vi "ProcesaDatos.vi"() -> ()   [LabVIEW 2010]
uses:
  <vilib>/Utility/file.llb/Write To Spreadsheet File (DBL).vi
panel:
  in  "Stimuli Offset":dbl=0.8
  out "rpm":dbl[](graph)=[-2.67, 1577.33, 1763.996667, 1773.996667, 1763.996667, 1770.663333, 1767.33, 1770.663333, 1770.663333, 1767.33, 1773.996667, 710.6633330000001, 39.350201999999996, -2.67, -2.67, -2.67, -2.67, -2.67, -2.67, -2.67]
  out "u_control":dbl[][](graph)=[[1.8699999999999999, 1.8699999999999999, 1.8699999999999999, 1.8699999999999999, 1.8699999999999999, 1.8699999999999999, 1.8699999999999999, 1.8699999999999999, 1.8699999999999999, 1.8699999999999999, -0.010000000000000009, -0.010000000000000009, -0.010000000000000009, -0.010000000000000009, -0.010000000000000009, -0.010000000000000009, -0.010000000000000009, -0.010000000000000009, -0.010000000000000009, -0.010000000000000009]]
  in  "Done":bool
  out "Signals":dbl[][](graph)=[[0.79, 0.79, 0.79, 0.79, 0.79, 0.79, 0.79, 0.79, 0.79, 0.79, 2.67, 2.67, 2.67, 2.67, 2.67, 2.67, 2.67, 2.67, 2.67, 2.67, 0.79, 0.79, 0.79, 0.79, 0.79, 0.79, 0.79, 0.79, 0.79, 0.79, 2.67, 2.67, 2.67, 2.67, 2.67, 2.67, 2.67, 2.67, 2.67, 2.67, 0.79, 0.79, 0.79, 0.79, 0.79, 0.79, 0.79, 0.79, 0.79, 0.79, 2.67, 2.67, 2.67, 2.67, 2.67, 2.67, 2.67, 2.67, 2.67, 2.67, 0.79, 0.79, 0.79, 0.79, 0.79], [0.0, 3.333333, 0.0, 0.0, 0.0, 0.0, 0.0, 0.0, 0.0, 0.0, 0.0, 1580.0, 1766.666667, 1776.666667, 1766.666667, 1773.333333, 1770.0, 1773.333333, 1773.333333, 1770.0, 1776.666667, 713.333333, 42.020202, 0.0, 0.0, 0.0, 0.0, 0.0, 0.0, 0.0, 0.0, 1583.333333, 1770.0, 1776.666667, 1770.0, 1773.333333, 1776.666667, 1770.0, 1776.666667, 1776.666667, 1773.333333, 713.333333, 20.0, 0.0, 0.0, 0.0, 0.0, 0.0, 0.0, 0.0, 0.0, 1583.333333, 1773.333333, 1776.666667, 1773.333333, 1773.333333, 1776.666667, 1773.333333, 1780.0, 1776.666667, 1776.666667, 713.333333, 50.0, 33.333333, 0.0]]
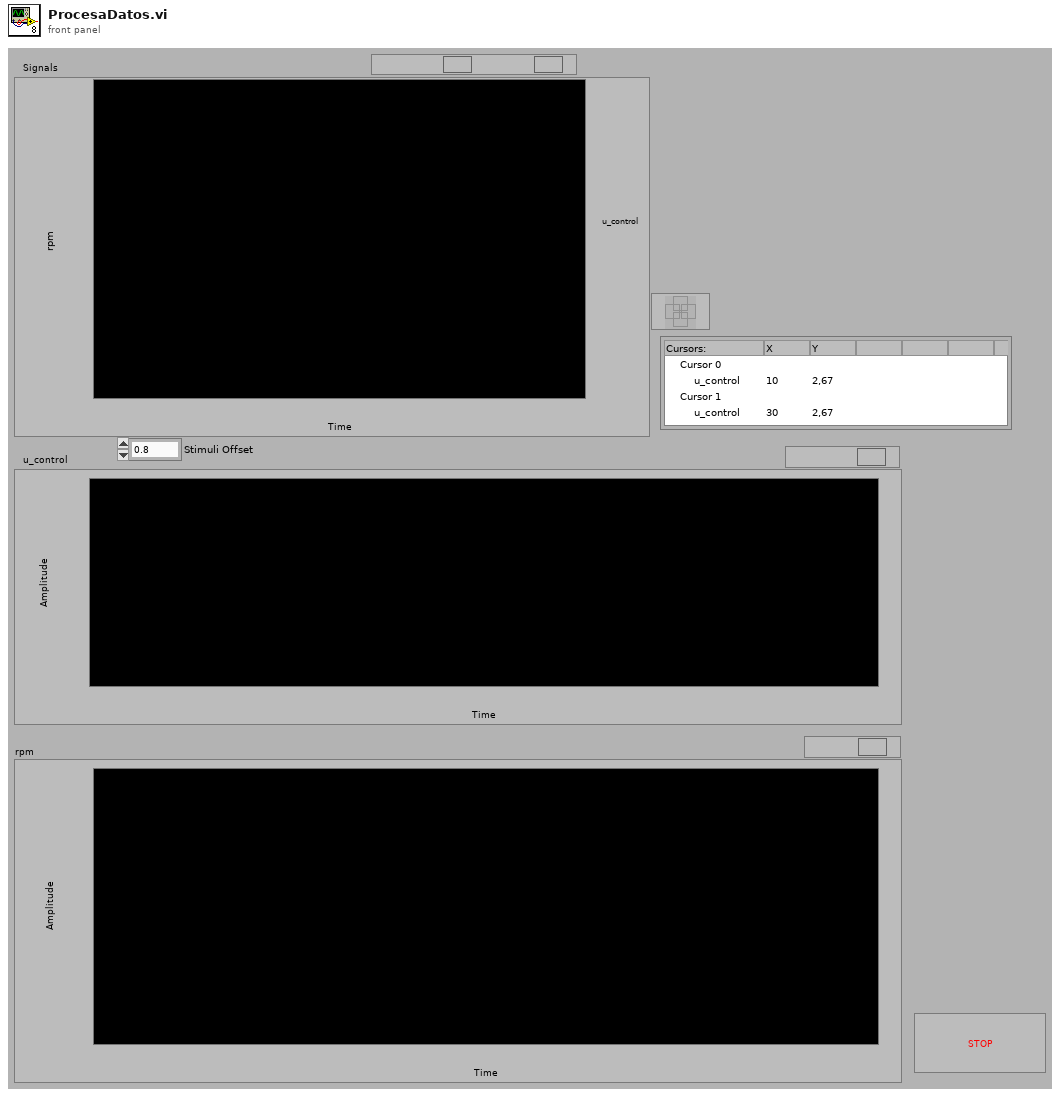
[diagram p1: front panel]
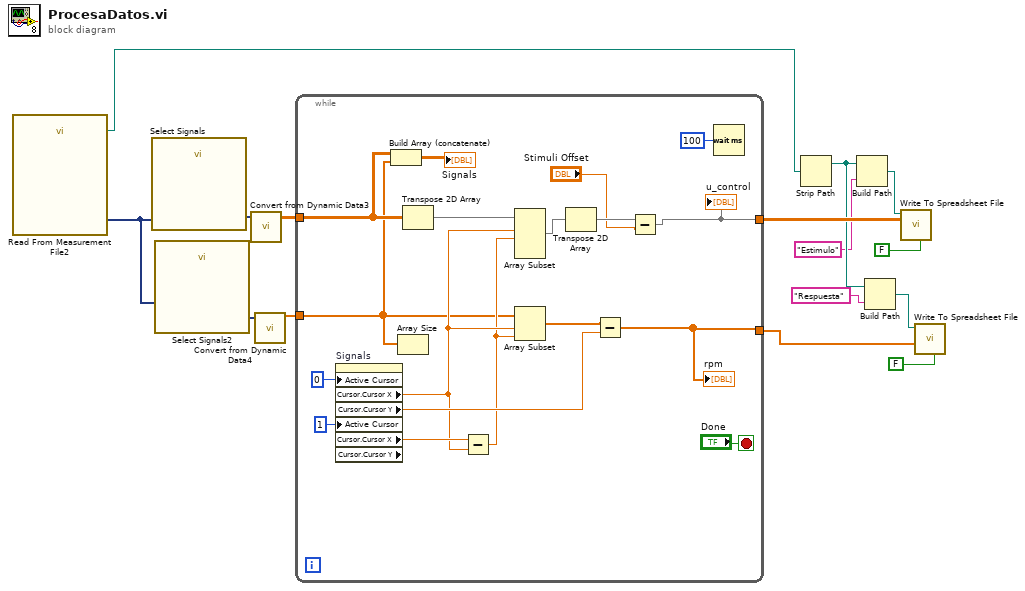
[diagram p0: block diagram]
diagram:
  n1 = call "Read From Measurement File2"() -> ("Filename Out"=w3:path, "Signals"=w15:dynamicdata)  [unwired: 6 in, 4 out]
  n2 = call "Select Signals"("Signals"=w15) -> ("Signal Out"=w14:dynamicdata)  [unwired: 2 in, 8 out]
  n3 = call "Select Signals2"("Signals"=w15) -> ("Signal Out"=w13:dynamicdata)  [unwired: 2 in, 8 out]
  n4 = call "Convert from Dynamic Data3"("Dynamic Data Type"=w14) -> ("Array"=w12:dbl[][])  [unwired: 3 out]
  n5 = call "Convert from Dynamic Data4"("Dynamic Data Type"=w13) -> ("Array"=w11:dbl[])  [unwired: 3 out]
  n6 = while {
    tunnel: w12 -> [w30]
    tunnel: w11 -> [w16]
    tunnel: [w25] -> w10
    tunnel: [w22] -> w9
    stop <- "Done" stop-if-true
    n7 = property on="Signals" class="WFGraph (strict)" props=["Active Cursor", "Cursor", "Cursor X", "Cursor", "Cursor Y", "Active Cursor", "Cursor", "Cursor X", "Cursor", "Cursor Y"]("Active Cursor"=u32 0, "Active Cursor"=u32 1) -> ("Cursor.Cursor X"=w18:dbl, "Cursor.Cursor Y"=w26:dbl, "Cursor.Cursor X"=w19:dbl)  [unwired: 2 in, 3 out]
    n8 = Build Array (concatenate)(w30, w16) -> (→"Signals":dbl[][])
    n9 = Array Size(array=w16) -> ()  [unwired: 1 out]
    n10 = Transpose 2D Array(2D array=w30) -> (transposed array=w29:dbl[][])
    n11 = Subtract(x=w19, y=w18) -> (x-y=w17:dbl)
    n12 = Array Subset(array=w29, index (row)=w18, length (row)=w17) -> (w28:dbl[][])  [unwired: 2 in]
    n13 = Array Subset(array=w16, index=w18, length=w17) -> (w27:dbl[])
    n14 = Transpose 2D Array(2D array=w28) -> (transposed array=w24:dbl[][])
    n15 = Subtract(x=w27, y=w26) -> (x-y=w25:dbl[])
    "rpm" <- w25
    n16 = Subtract(x=w24, y="Stimuli Offset") -> (x-y=w22:dbl[][])
    "u_control" <- w22
    n17 = Wait (ms)(milliseconds to wait=u32 100) -> ()  [unwired: 1 out]
  }
  n18 = Strip Path(path=w3) -> (stripped path=w8:path)  [unwired: 1 out]
  n19 = Build Path(base path=w8, name or relative path="Estimulo") -> (appended path=w5:path)
  n20 = Build Path(base path=w8, name or relative path="Respuesta") -> (appended path=w4:path)
  n21 = call-poly <vilib>:"Write To Spreadsheet File.vi"("transpose? (no:F)"=FALSE, "2D data"=w9, "file path (dialog if empty)"=w5) -> ()  [unwired: 3 in, 3 out]
  n22 = call-poly <vilib>:"Write To Spreadsheet File.vi"("transpose? (no:F)"=FALSE, "1D data"=w10, "file path (dialog if empty)"=w4) -> ()  [unwired: 3 in, 3 out]
